vi "Read Exit.vi"(8 "error in (no error)":errorcluster, 11 "AbstractionMessage in":refnum<class "AbstractionMessage.lvclass">) -> (0 "error out":errorcluster, 2 "Exit":bool, 3 "AbstractionMessage out":refnum<class "AbstractionMessage.lvclass">)   [LabVIEW 2021, in "AbstractionMessage.lvclass"]
uses:
  AbstractionMessage.lvclass
  AbstractionMessage.lvclass/AbstractionMessage.ctl
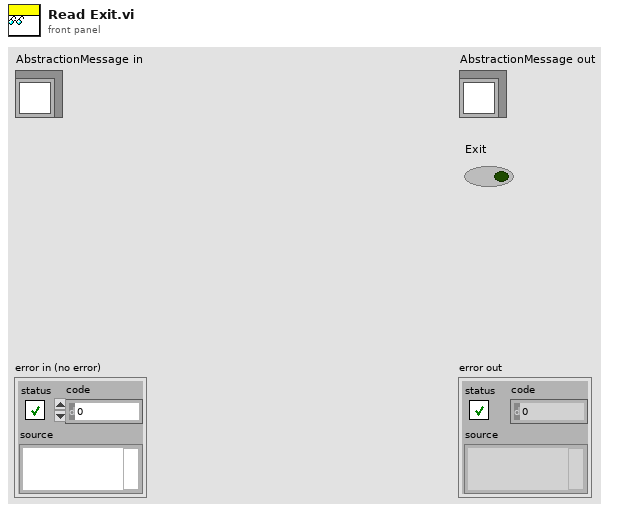
[diagram p1: front panel]
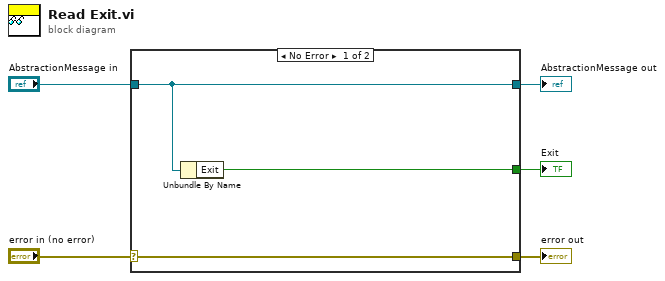
[diagram p0: block diagram]
diagram:
  n1 = case shown="No Error" "error in (no error)" {
    selector: "error in (no error)" -> [w8 w9]
    tunnel: [w8 w9] -> w4
    tunnel: [w7 w10] -> w2
    tunnel: "AbstractionMessage in" -> [w7 w10]
    tunnel: [w6 _] -> w1
    frame No Error {
      n2 = Unbundle By Name(w7) -> ("Exit"=w6:bool)
    }
    frame Error {
    }
  }
  "error out" <- w4
  "AbstractionMessage out" <- w2
  "Exit" <- w1
